vi "2D Wave PDE Rendering (Rect Domain).vi"(0 "PDE in":refnum<class "NI_PDE.lvclass">, 5 "U(t, x, y)":dbl[][][](array[numeric]), 7 "index (time step)":i32=-1, 11 "error in (no error)":errorcluster) -> (4 "PDE out":refnum<class "NI_PDE.lvclass">, 6 "PDE Plot":dbl[][](graph), 8 "X Scale":T1, 10 "Y Scale":T1, 15 "error out":errorcluster)   [LabVIEW 2020, in "NI_PDE.lvlib"]
doc: "Renders the solution of the partial differential equation. You must manually select the polymorphic instance to use."
uses:
  <vilib>/gmath/NI_PDE.lvlib
  <vilib>/gmath/pde.llb/PDEClass/NI_PDE.lvclass
  <vilib>/Utility/miscctls.llb/LVOffsetAndMultiplierTypeDef.ctl
  <vilib>/gmath/pde.llb/DomainClass/Domain_Evolut_2D_Rect/NI_Domain_Evolut_2D_Rect.lvclass
  e:/builds/penguin/labview/branches/2020/dev/dist/vi.lib/gmath/pde.llb/DomainClass/NI_Domain.lvclass
  <vilib>/gmath/pde.llb/PDEClass/PDE_Wave_2D/NI_PDE_Wave_2D.lvclass
  e:/builds/penguin/labview/branches/2020/dev/dist/vi.lib/gmath/pde.llb/PDEClass/NI_PDE.lvclass
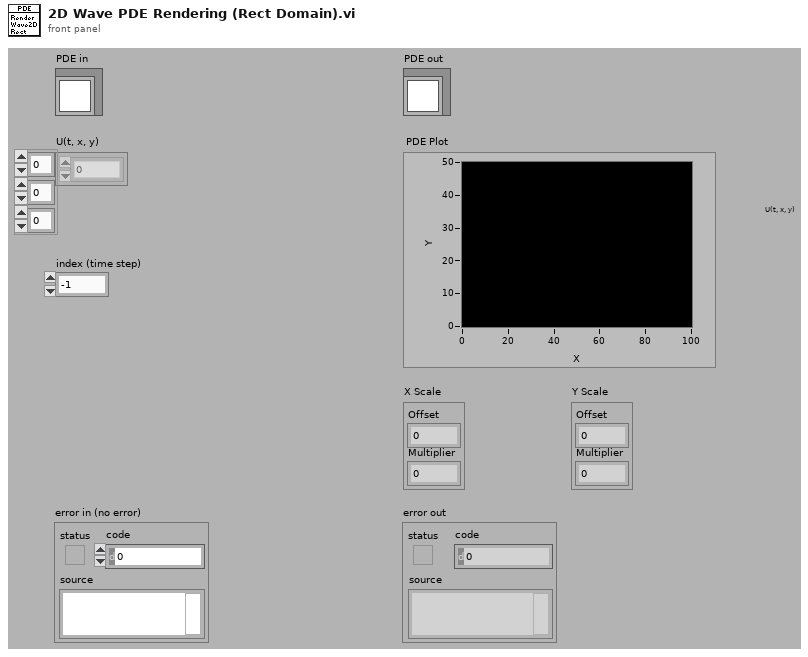
[diagram p1: front panel]
types:
  T1 = typedef "LVOffsetAndMultiplierTypeDef.ctl" = cluster{"Offset":dbl, "Multiplier":dbl}
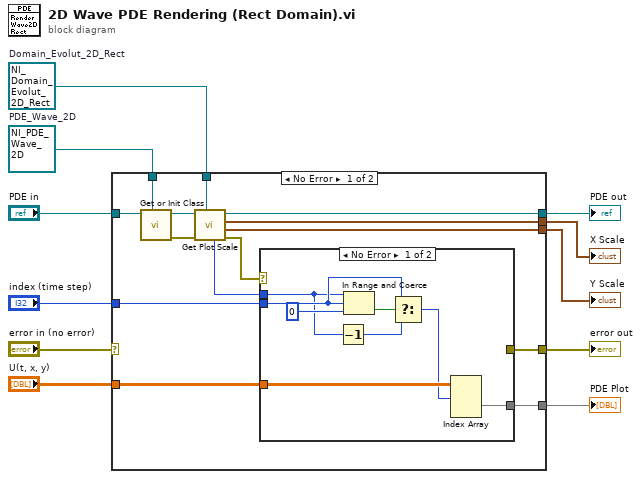
[diagram p0: block diagram]
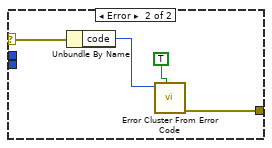
[diagram p2: hidden frame]
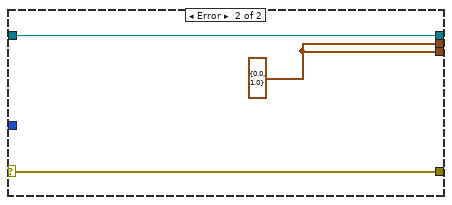
[diagram p3: hidden frame]
diagram:
  w1 = refnum<class "NI_PDE_Wave_2D.lvclass"> refnum  # PDE_Wave_2D
  w2 = refnum<class "NI_Domain_Evolut_2D_Rect.lvclass"> refnum  # Domain_Evolut_2D_Rect
  n1 = case shown="No Error" "error in (no error)" {
    selector: "error in (no error)" -> [_ w39]
    tunnel: "U(t, x, y)" -> [w25 _]
    tunnel: [w24 _] -> w10
    tunnel: "index (time step)" -> [w23 _]
    tunnel: [w18 w40] -> w8
    tunnel: [w17 w38] -> w7
    tunnel: [w16 w38] -> w6
    tunnel: "PDE in" -> [w19 w40]
    tunnel: [w22 w39] -> w4
    tunnel: w2 -> [w13 _]
    tunnel: w1 -> [w12 _]
    frame No Error {
      n2 = call <vilib>:"Get or Init Class.vi"("target PDE"=w12, "PDE in"=w19) -> ("error out"=w20:errorcluster, "PDE out"=w21:refnum<class "NI_PDE.lvclass">)  [unwired: 1 in, 7 out]
      n3 = call <vilib>:"Get Plot Scale.vi"("target Domain"=w13, "error in (no error)"=w20, "PDE in"=w21) -> ("error out"=w15:errorcluster, "Y Scale"=w16:T1, "X Scale"=w17:T1, "PDE out"=w18:refnum<class "NI_PDE.lvclass">, "# of t-points"=w14:i32)  [unwired: 4 out]
      n4 = case shown="No Error" w15 {
        selector: w15 -> [_ w35]
        tunnel: w25 -> [w31 _]
        tunnel: [w30 _] -> w24
        tunnel: w23 -> [w27 _]
        tunnel: w14 -> [w26 _]
        tunnel: [_ w34] -> w22
        frame No Error {
          n5 = Decrement(x=w26) -> (x-1=w28:i32)
          n6 = In Range and Coerce(upper limit=w26, x=w27, lower limit=0) -> (In Range?=w32:bool)  [unwired: 1 out]
          n7 = Select(t=w27, s=w32, f=w28) -> (s? t:f=w29:i32)
          n8 = Index Array(array=w31, index (dim 0)=w29) -> (element=w30:dbl[][])  [unwired: 2 in]
        }
        frame Error {
          n9 = Unbundle By Name(w35) -> ("code"=w37:i32)
          n10 = call <vilib>:"Error Cluster From Error Code.vi"("show call chain? (False)"=TRUE, "error code (0)"=w37) -> ("error out"=w34:errorcluster)  [unwired: 1 in, 6 out]
        }
      }
    }
    frame Error {
      w38 = T1 {"Offset"=0.0, "Multiplier"=1.0} ("Offset and Multiplier")
    }
  }
  "PDE out" <- w8
  "error out" <- w4
  "PDE Plot" <- w10
  "X Scale" <- w7
  "Y Scale" <- w6
